vi "Yokogawa Class Chooser Real.vi"(11 "Incoming ID in":string="\n") -> (0 "Enum":T1=enum."WT500", 1 "Model":string, 3 "Universal Power Meter out":refnum<class "Universal Power Meter.lvclass">)   [LabVIEW 2013, in "Universal Power Meter.lvlib" / "Universal Power Meter.lvclass"]
uses:
  Universal Power Meter.lvclass
  Models.ctl
  Yokogawa WT500/Yokogawa WT500.lvclass
  Yokogawa WT2X0/Yokogawa WT2X0.lvclass
  Yokogawa WT1600/Yokogawa WT1600.lvclass
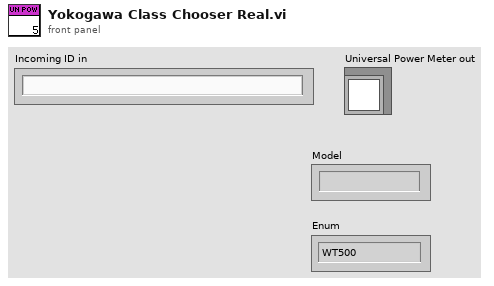
[diagram p1: front panel]
types:
  T1 = typedef "Universal Power Meter.lvlib/Universal Power Meter.lvclass/Models.ctl" = enum16{"Unknown", "WT500", "WT1600", "WT230", "WT210"}
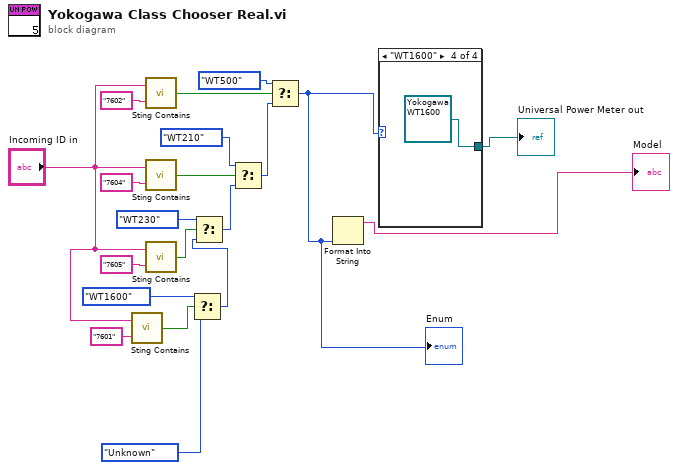
[diagram p0: block diagram]
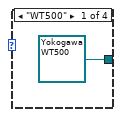
[diagram p2: hidden frame]
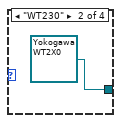
[diagram p3: hidden frame]
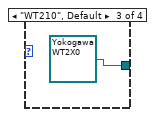
[diagram p4: hidden frame]
diagram:
  n1 = call "Sting Contains.vi"("Expression to evaluate"="7601", "Input String"="Incoming ID in") -> ("String Contains?"=w5:bool)
  n2 = call "Sting Contains.vi"("Expression to evaluate"="7602", "Input String"="Incoming ID in") -> ("String Contains?"=w17:bool)
  n3 = call "Sting Contains.vi"("Expression to evaluate"="7604", "Input String"="Incoming ID in") -> ("String Contains?"=w16:bool)
  n4 = call "Sting Contains.vi"("Expression to evaluate"="7605", "Input String"="Incoming ID in") -> ("String Contains?"=w14:bool)
  n5 = Select(t=Models."WT1600" ("Enum"), s=w5, f=Models."Unknown" ("Enum")) -> (s? t:f=w2:T1)
  n6 = Select(t=Models."WT230" ("Enum"), s=w14, f=w2) -> (s? t:f=w13:T1)
  n7 = Select(t=Models."WT210" ("Enum"), s=w16, f=w13) -> (s? t:f=w15:T1)
  n8 = Select(t=Models."WT500" ("Enum"), s=w17, f=w15) -> (s? t:f=w1:T1)
  "Enum" <- w1
  n9 = Format Into String(w1) -> (resulting string=→"Model":string)  [unwired: 3 in, 1 out]
  n10 = case shown="\"WT1600\"" w1 {
    tunnel: [refnum<class "Yokogawa WT500.lvclass"> refnum ("Universal Power Meter.lvlib:Yokogawa WT500.lvlib:Yokogawa WT500.lvclass") refnum<class "Yokogawa WT2X0.lvclass"> refnum ("Universal Power Meter.lvlib:Yokogawa WT2X0.lvlib:Yokogawa WT2X0.lvclass") refnum<class "Yokogawa WT2X0.lvclass"> refnum ("Universal Power Meter.lvlib:Yokogawa WT2X0.lvlib:Yokogawa WT2X0.lvclass") refnum<class "Yokogawa WT1600.lvclass"> refnum ("Universal Power Meter.lvlib:Yokogawa WT1600.lvlib:Yokogawa WT1600.lvclass")] -> w9
    frame "WT500" {
    }
    frame "WT230" {
    }
    frame "WT210", Default {
    }
    frame "WT1600" {
    }
  }
  "Universal Power Meter out" <- w9
